vi "New.vi"(8 "error in (no error)":errorcluster, 10 "timeout":i32=10000, 11 "Socket.UDP in":refnum<class "Socket.UDP.lvclass">) -> (0 "error out":errorcluster, 3 "Socket.UDP out":refnum<class "Socket.UDP.lvclass">)   [LabVIEW 2014, in "Socket.lvlib" / "Socket.UDP.lvclass"]
doc: "Creates a new socket object. Sets the timeout and \"initialized\" property."
uses:
  Socket.UDP.lvclass
  Socket.Base/Socket.Base.lvclass
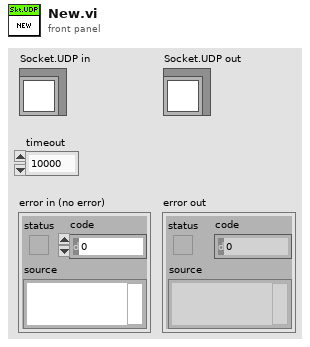
[diagram p1: front panel]
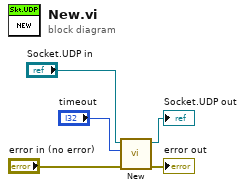
[diagram p0: block diagram]
diagram:
  n1 = call-parent "New.vi"("error in (no error)"="error in (no error)", "timeout"="timeout", "Socket.Base in"="Socket.UDP in") -> ("error out"=→"error out":errorcluster, "Socket.Base out"=→"Socket.UDP out":refnum<class "Socket.UDP.lvclass">)  [unwired: 7 in]
